vi "solar_misc Email Send.vi"(0 "Recipients":string[](array[string]), 1 "Mail Server (\"mail.aero.ball.com\")":string="mail.aero.ball.com", 2 "Mail Server Port (25)":u16=25, 5 "Subject":string="[No Subject]", 7 "Message":string="This is a test", 9 "Return Address":string="batcsolar@ball.com", 11 "error in (no error)":errorcluster, 12 "TCP Timeout (5000ms)":i32=5000) -> (8 "All Responses Valid?":bool, 10 "Response Codes":i32[](array[numeric]), 15 "error out":errorcluster)   [LabVIEW 2018]
doc: "This VI sends an email."
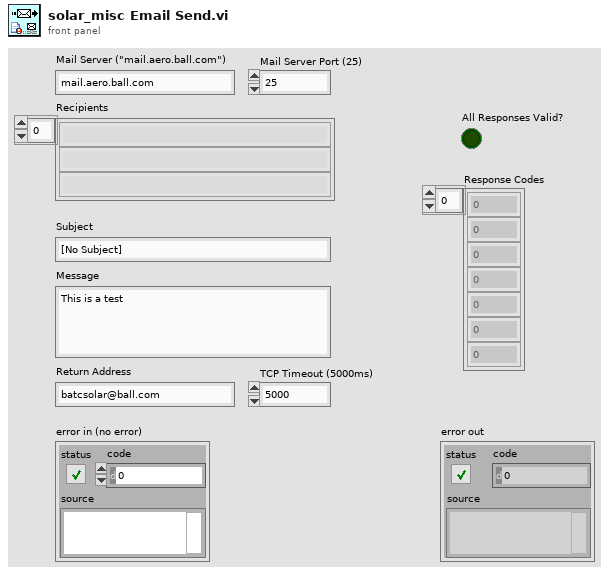
[diagram p1: front panel]
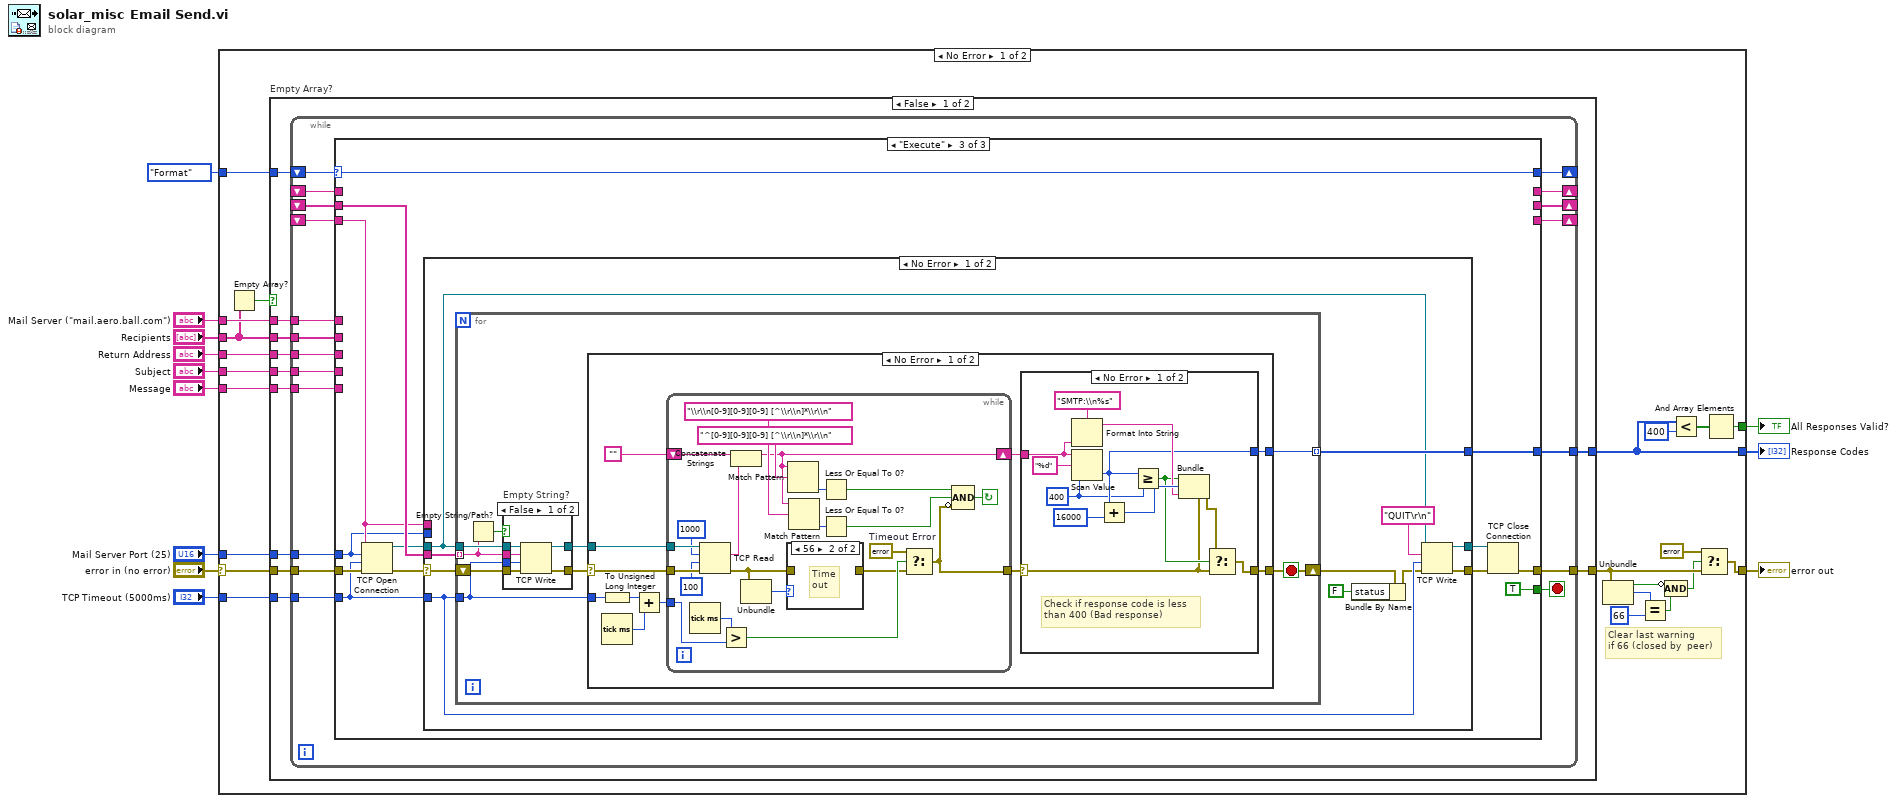
[diagram p0: block diagram]
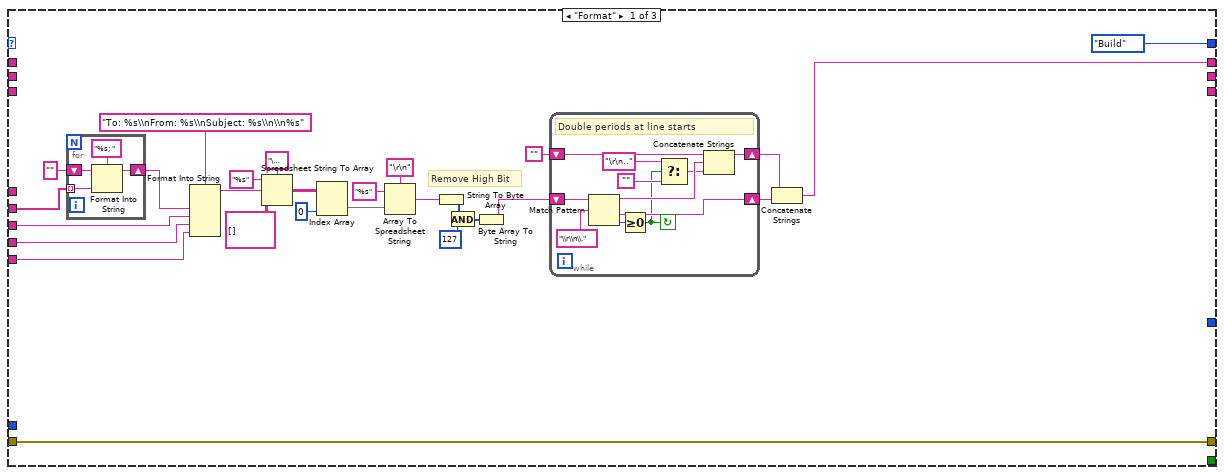
[diagram p2: hidden frame]
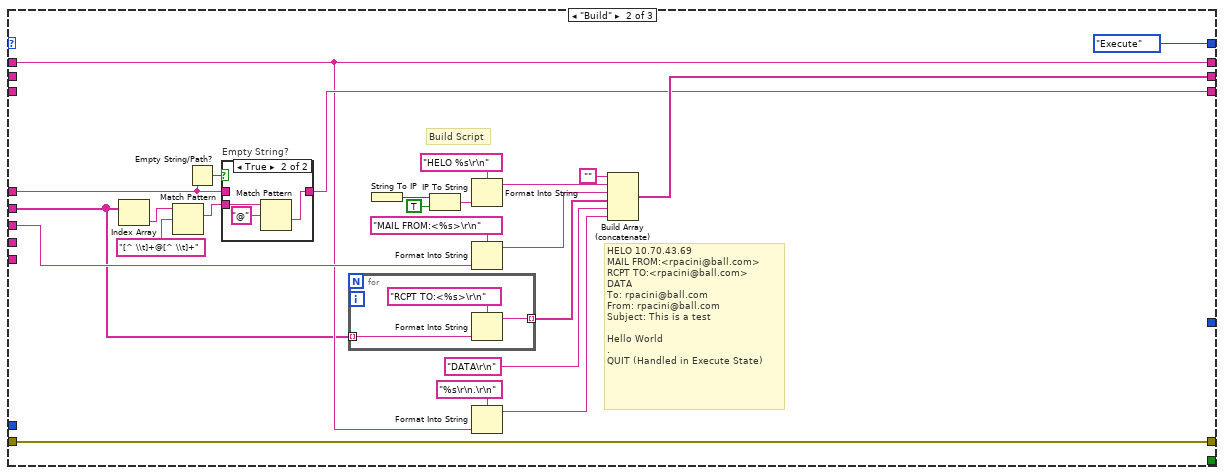
[diagram p3: hidden frame]
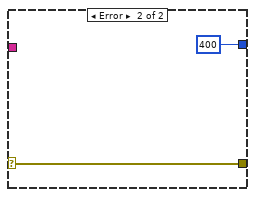
[diagram p7: hidden frame]
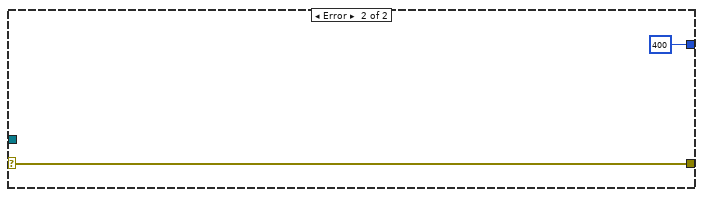
[diagram p8: hidden frame]
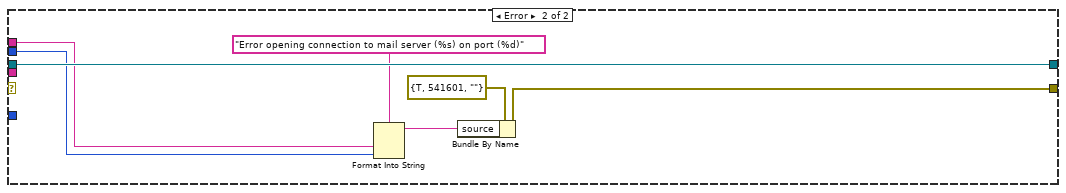
[diagram p9: hidden frame]
diagram:
  n1 = case shown="No Error" "error in (no error)" {
    selector: "error in (no error)" -> [w34 w237]
    tunnel: [w19 w237] -> w4
    tunnel: "TCP Timeout (5000ms)" -> [w33 _]
    tunnel: "Message" -> [w32 _]
    tunnel: "Subject" -> [w31 _]
    tunnel: "Return Address" -> [w30 _]
    tunnel: "Recipients" -> [w14 _]
    tunnel: "Mail Server (\"mail.aero.ball.com\")" -> [w29 _]
    tunnel: "Mail Server Port (25)" -> [w28 _]
    tunnel: enum16{"Format", "Build", "Execute"}."Format" -> [w27 _]
    tunnel: [w18 _] -> w2
    tunnel: [w15 _] -> w1
    frame No Error {
      # "Clear last warning\nif 66 (closed by  peer)"
      n2 = Empty Array?(array=w14) -> (empty?=w13:bool)
      n3 = case "Empty Array?" shown="False" w13 {
        tunnel: w34 -> [w45 w236]
        tunnel: w33 -> [w44 _]
        tunnel: w32 -> [w43 _]
        tunnel: w31 -> [w42 _]
        tunnel: w30 -> [w41 _]
        tunnel: w29 -> [w40 _]
        tunnel: w28 -> [w39 _]
        tunnel: w27 -> [w38 _]
        tunnel: [w37 w236] -> w24
        tunnel: [w36 _] -> w18
        tunnel: w14 -> [w35 _]
        frame False {
          n4 = while {
            tunnel: w45 -> [w64]
            tunnel: [w63] -> w37
            tunnel: w44 -> [w62]
            tunnel: w43 -> [w61]
            tunnel: w42 -> [w60]
            tunnel: w41 -> [w59]
            tunnel: w35 -> [w58]
            shift-right: [w57] -> _
            shift-left: _ -> [w56]
            shift-right: [w55] -> _
            shift-left: _ -> [w54]
            shift-right: [w53] -> _
            shift-left: _ -> [w52]
            tunnel: w40 -> [w51]
            tunnel: w39 -> [w49]
            shift-right: [w47] -> _
            shift-left: w38 -> [w48]
            tunnel: [w46] -> w36
            stop <- w50 stop-if-true
            n5 = case shown="\"Execute\"" w48 {
              tunnel: [w72 w110 w150] -> w63
              tunnel: w64 -> [w72 w110 w148]
              tunnel: w62 -> [_ _ w140]
              tunnel: w61 -> [w77 _ _]
              tunnel: w60 -> [w76 _ _]
              tunnel: w59 -> [w75 w117 _]
              tunnel: w58 -> [w69 w107 _]
              tunnel: [_ w114 _] -> w57
              tunnel: w56 -> [_ _ w147]
              tunnel: [_ w113 _] -> w55
              tunnel: w54 -> [_ _ w139]
              tunnel: [w74 w112 _] -> w53
              tunnel: w52 -> [_ w112 _]
              selector: w48 -> [_ _ w145]
              tunnel: w51 -> [_ w111 _]
              tunnel: [_ _ TRUE] -> w50
              tunnel: w49 -> [_ _ w138]
              tunnel: [enum16{"Format", "Build", "Execute"}."Build" enum16{"Format", "Build", "Execute"}."Execute" w145] -> w47
              tunnel: [_ _ w144] -> w46
              frame "Format" {
                # "Remove High Bit"
                n6 = for {
                  tunnel: w69 -> [w95] mode=indexing
                  shift-right: [w93] -> w68
                  shift-left: "" -> [w92]
                  n7 = Format Into String(format string="%s; ", initial string=w92, w95) -> (resulting string=w93:string)  [unwired: 1 in, 1 out]
                }
                n8 = Format Into String(format string="To: %s\\nFrom: %s\\nSubject: %s\\n\\n%s", w68, w75, w76, w77) -> (resulting string=w83:string)  [unwired: 2 in, 1 out]
                n9 = Spreadsheet String To Array(delimiter (Tab)="\u0000", format string="%s", spreadsheet string=w83, array type (2D Dbl)=string[][] []) -> (array=w88:string[][])
                n10 = Index Array(array=w88, index (col)=0 ("disabled index (col)")) -> (element=w85:string[])  [unwired: 1 in]
                n11 = Array To Spreadsheet String(delimiter (Tab)="\r\n", array=w85, 3:"%s" ("format string")) -> (spreadsheet string=w82:string)
                n12 = String To Byte Array(string=w82) -> (unsigned byte array=w65:u8[])
                n13 = And(x=w65, y=u8 127) -> (x .and. y?=w67:u8[])
                n14 = Byte Array To String(unsigned byte array=w67) -> (string=w78:string)
                n15 = while {
                  shift-left: w78 -> [w100]
                  shift-right: [w99] -> w79
                  shift-left: "" -> [w106]
                  shift-right: [w105] -> w80
                  stop <- w96 continue-if-true
                  # "Double periods at line starts"
                  n16 = Match Pattern(string=w100, regular expression="\\r\\n\\.") -> (before substring=w104:string, after substring=w99:string, offset past match=w103:i32)  [unwired: 1 in, 1 out]
                  n17 = Greater Or Equal To 0?(x=w103) -> (x >= 0?=w96:bool)
                  n18 = Select(t="\r\n.." ("regular expression"), s=w96, f="") -> (s? t:f=w102:string)
                  n19 = Concatenate Strings(w106, w104, w102) -> (w105:string)
                }
                n20 = Concatenate Strings(w80, w79) -> (w74:string)
              }
              frame "Build" {
                # "HELO 10.70.43.69\nMAIL FROM:<rpacini@ball.com>\nRCPT TO:<rpacini@ball.com>\nDATA\nTo: rpacini@ball.com\nFrom: rpacini@ball.com\nSubject: This is a test\n\nHello World\n.\nQUIT (Handled in Execute State)"
                # "Build Script"
                n21 = Index Array(array=w107) -> (element=w108:string)  [unwired: 1 in]
                n22 = Match Pattern(string=w108, regular expression="[^ \\t]+@[^ \\t]+") -> (match substring=w115:string)  [unwired: 1 in, 3 out]
                n23 = Empty String/Path?(string/path=w111) -> (empty?=w118:bool)
                n24 = case "Empty String?" shown="True" w118 {
                  tunnel: w115 -> [_ w137]
                  tunnel: [w134 w135] -> w113
                  tunnel: w111 -> [w134 _]
                  frame False {
                  }
                  frame True {
                    n25 = Match Pattern(string=w137, regular expression="@") -> (after substring=w135:string)  [unwired: 1 in, 3 out]
                  }
                }
                n26 = for {
                  tunnel: [w133] -> w127 mode=indexing
                  tunnel: w107 -> [w131] mode=indexing
                  n27 = Format Into String(format string="RCPT TO:<%s>\r\n", w131) -> (resulting string=w133:string)  [unwired: 2 in, 1 out]
                }
                n28 = String To IP() -> (0:w122:u32)  [unwired: 1 in]
                n29 = IP To String(1:TRUE ("dot notation? (F)"), 2:w122) -> (0:w120:string)
                n30 = Format Into String(format string="HELO %s\r\n", w120) -> (resulting string=w123:string)  [unwired: 2 in, 1 out]
                n31 = Format Into String(format string="MAIL FROM:<%s>\r\n", w117) -> (resulting string=w126:string)  [unwired: 2 in, 1 out]
                n32 = Format Into String(format string="%s\r\n.\r\n", w112) -> (resulting string=w130:string)  [unwired: 2 in, 1 out]
                n33 = Build Array (concatenate)("", w123, w126, w127, "DATA\r\n", w130) -> (w114:string[])
              }
              frame "Execute" {
                n34 = TCP Open Connection(address=w139, remote port or service name=w138, timeout ms (60000)=w140, error in (no error)=w148) -> (connection ID=w142:refnum<k5>, error out=w149:errorcluster)  [unwired: 1 in]
                n35 = case shown="No Error" w149 {
                  selector: w149 -> [w161 _]
                  tunnel: w147 -> [w160 _]
                  tunnel: [w159 _] -> w144
                  tunnel: [w158 w229] -> w143
                  tunnel: w142 -> [w156 w235]
                  tunnel: [w155 w235] -> w141
                  tunnel: w140 -> [w154 _]
                  tunnel: w139 -> [_ w233]
                  tunnel: w138 -> [_ w232]
                  frame No Error {
                    n36 = for {
                      shift-right: [w162] -> w152
                      shift-left: w161 -> [w170]
                      tunnel: w156 -> [w169]
                      tunnel: w160 -> [w168] mode=indexing
                      tunnel: w154 -> [w167]
                      tunnel: [w166] -> w159 mode=indexing
                      stop <- w162 stop-if-true
                      n37 = Empty String/Path?(string/path=w168) -> (empty?=w163:bool)
                      n38 = case "Empty String?" shown="False" w163 {
                        tunnel: [w176 w177] -> w164
                        tunnel: w168 -> [w175 _]
                        tunnel: [w174 w178] -> w165
                        tunnel: w169 -> [w173 w178]
                        tunnel: w170 -> [w172 w177]
                        tunnel: w167 -> [w171 _]
                        frame False {
                          n39 = TCP Write(connection ID=w173, data in=w175, error in (no error)=w172, 9:w171) -> (connection ID out=w174:refnum<k5>, error out=w176:errorcluster)  [unwired: 1 out]
                        }
                        frame True {
                        }
                      }
                      n40 = case shown="No Error" w164 {
                        selector: w164 -> [w187 w228]
                        tunnel: [w185 w228] -> w162
                        tunnel: w165 -> [w188 _]
                        tunnel: w167 -> [w182 _]
                        tunnel: [w179 400 ("bytes to read")] -> w166
                        frame No Error {
                          n41 = To Unsigned Long Integer(number=w182) -> (unsigned 32bit integer=w181:u32)
                          n42 = Tick Count (ms)() -> (millisecond timer value=w183:u32)
                          n43 = Add(x=w181, y=w183) -> (x+y=w180:u32)
                          n44 = while {
                            shift-left: "" -> [w207]
                            shift-right: [w198] -> w184
                            tunnel: w187 -> [w210]
                            tunnel: [w190] -> w186
                            tunnel: w188 -> [w211]
                            tunnel: w180 -> [w196]
                            stop <- w202 continue-if-true
                            w194 = errorcluster {"status"=TRUE, "code"=5056, "source"="SMTP: Response Timeout"}  # Timeout Error
                            n45 = Tick Count (ms)() -> (millisecond timer value=w197:u32)
                            n46 = TCP Read(connection ID=w211, bytes to read=1000, error in (no error)=w210, 9:100 ("bytes to read")) -> (data out=w206:string, error out=w192:errorcluster)  [unwired: 1 in, 1 out]
                            n47 = Greater?(x=w197, y=w196) -> (0:w195:bool)
                            n48 = Concatenate Strings(w207, w206) -> (w198:string)
                            n49 = Unbundle(w192) -> ("code"=w193:i32)  [unwired: 2 out]
                            n50 = case shown="56" w193 {
                              tunnel: w192 -> [w212 _]
                              tunnel: [w212 _] -> w191
                              frame Default {
                              }
                              frame 56 {
                                # "Time\nout"
                              }
                            }
                            n51 = Match Pattern(string=w198, regular expression="^[0-9][0-9][0-9] [^\\r\\n]*\\r\\n") -> (offset past match=w204:i32)  [unwired: 1 in, 3 out]
                            n52 = Match Pattern(string=w198, regular expression="\\r\\n[0-9][0-9][0-9] [^\\r\\n]*\\r\\n") -> (offset past match=w201:i32)  [unwired: 1 in, 3 out]
                            n53 = Less Or Equal To 0?(x=w204) -> (x <= 0?=w203:bool)
                            n54 = Less Or Equal To 0?(x=w201) -> (x <= 0?=w200:bool)
                            n55 = Select(t=w194, s=w195, f=w191) -> (s? t:f=w190:errorcluster)
                            n56 = Compound Arithmetic op=AND(w203, w200, invert w190) -> (w202:bool)
                          }
                          n57 = case shown="No Error" w186 {
                            selector: w186 -> [w216 w226]
                            tunnel: [w215 w226] -> w185
                            tunnel: w184 -> [w221 _]
                            tunnel: [w214 400 ("bytes to read")] -> w179
                            frame No Error {
                              w213 = 400 ("bytes to read")
                              # "Check if response code is less\nthan 400 (Bad response)"
                              n58 = Format Into String(format string="SMTP:\\n%s", w221) -> (resulting string=w220:string)  [unwired: 2 in, 1 out]
                              n59 = Scan Value(string=w221, format string="%d", default (0 dbl)=w213) -> (value=w214:i32)  [unwired: 1 out]
                              n60 = Add(x=w214, y=16000) -> (x+y=w222:i32)
                              n61 = Greater Or Equal?(x=w214, y=w213) -> (x >= y?=w218:bool)
                              n62 = Bundle(cluster=w216, "status"=w218, "code"=w222, "source"=w220) -> (w217:errorcluster)
                              n63 = Select(t=w217, s=w218, f=w216) -> (s? t:f=w215:errorcluster)
                            }
                            frame Error {
                            }
                          }
                        }
                        frame Error {
                        }
                      }
                    }
                    n64 = Bundle By Name(cluster=w152, "status"=FALSE) -> (w151:errorcluster)
                    n65 = TCP Write(connection ID=w156, data in="QUIT\r\n", error in (no error)=w151, 9:w154) -> (connection ID out=w155:refnum<k5>, error out=w158:errorcluster)  [unwired: 1 out]
                  }
                  frame Error {
                    n66 = Format Into String(format string="Error opening connection to mail server (%s) on port (%d)" ("source"), w233, w232) -> (resulting string=w230:string)  [unwired: 2 in, 1 out]
                    n67 = Bundle By Name(cluster=errorcluster {"status"=TRUE, "code"=541601, "source"=""} ("error IO"), "source"=w230) -> (w229:errorcluster)
                  }
                }
                n68 = TCP Close Connection(connection ID=w141, error in (no error)=w143) -> (error out=w150:errorcluster)  [unwired: 1 in, 1 out]
              }
            }
          }
        }
        frame True {
        }
      }
      n69 = Unbundle(w24) -> ("status"=w22:bool, "code"=w26:i32)  [unwired: 1 out]
      n70 = Equal?(x=w26, y=66) -> (x = y?=w23:bool)
      n71 = Compound Arithmetic op=AND(invert w22, w23) -> (w21:bool)
      n72 = Less?(x=w18, y=400) -> (x < y?=w16:bool[])
      n73 = Select(t=errorcluster {"status"=FALSE, "code"=0, "source"=""}, s=w21, f=w24) -> (s? t:f=w19:errorcluster)
      n74 = And Array Elements(Boolean array=w16) -> (logical AND=w15:bool)
    }
    frame Error {
    }
  }
  "error out" <- w4
  "Response Codes" <- w2
  "All Responses Valid?" <- w1
